vi "oa_Calculate Max Axis Display Value.vi"(9 "max axis display value in":dbl, 10 "orbit data Y":dbl[](array[numeric]), 11 "orbit data X":dbl[](array[numeric])) -> (3 "max data value out":dbl)   [LabVIEW 2017]
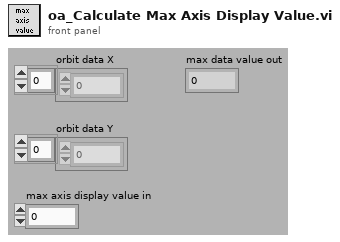
[diagram p1: front panel]
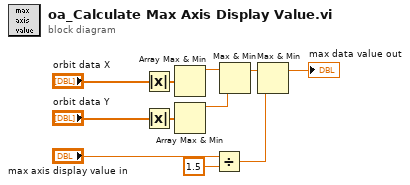
[diagram p0: block diagram]
diagram:
  n1 = Absolute Value(x="orbit data X") -> (abs(x)=w5:dbl[])
  n2 = Absolute Value(x="orbit data Y") -> (abs(x)=w6:dbl[])
  n3 = Array Max & Min(array=w5) -> (max value=w3:dbl)  [unwired: 3 out]
  n4 = Array Max & Min(array=w6) -> (max value=w4:dbl)  [unwired: 3 out]
  n5 = Divide(x="max axis display value in", y=1.5) -> (x/y=w9:dbl)
  n6 = Max & Min(x=w3, y=w4) -> (max(x,y)=w8:dbl)  [unwired: 1 out]
  n7 = Max & Min(x=w8, y=w9) -> (max(x,y)=→"max data value out":dbl)  [unwired: 1 out]
